vi "AddIfTrue.vi"(9 "To Add":refnum<class "Action.lvclass">[](array[class]), 10 "True?":bool, 11 "ActionStack in":refnum<class "Action.lvclass">[](array[class])) -> (3 "ActionStack out":refnum<class "Action.lvclass">[](array[class]))   [LabVIEW 2024, in "ActionStack.lvlib" / "Action.lvclass"]
uses:
  Action.lvclass
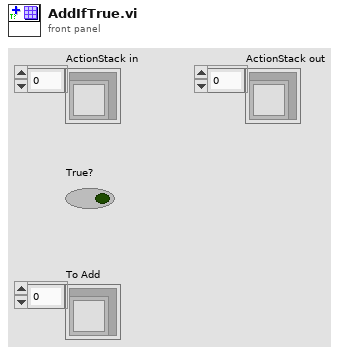
[diagram p1: front panel]
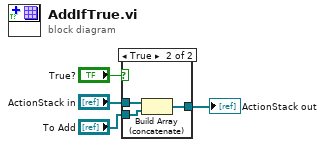
[diagram p0: block diagram]
diagram:
  n1 = case shown="True" "True?" {
    tunnel: [w5 w8] -> w4
    tunnel: "ActionStack in" -> [w5 w7]
    tunnel: "To Add" -> [_ w6]
    frame False {
    }
    frame True {
      n2 = Build Array (concatenate)(w7, w6) -> (w8:refnum<class "Action.lvclass">[])
    }
  }
  "ActionStack out" <- w4
